vi "Show Panel.vi"(8 "error in (no error)":errorcluster, 11 "View In":refnum<class "View.lvclass">) -> (0 "error out":errorcluster, 3 "View Out":refnum<class "View.lvclass">)   [LabVIEW 2020, in "View.lvclass"]
doc: "Show the front panel of the View."
uses:
  View.lvclass
  C:/Users/anton/Documents/GitHub/Triarc-Framework/source/Framework/Process/Process.lvclass
  Process/Process.lvclass/Process.ctl
  View.lvclass/View.ctl
  Process/Public/Get Lifecycle State.vi
  Process/Protected/Messaging/Request Message.vi
  <vilib>/Utility/error.llb/Clear Errors.vi
  Process/Private/SubVIs/Enqueue Request Message.vi
  <vilib>/Utility/error.llb/Error Cluster From Error Code.vi
  Process/Private/SubVIs/Wait for Response Message.vi
  Process/Process.lvclass
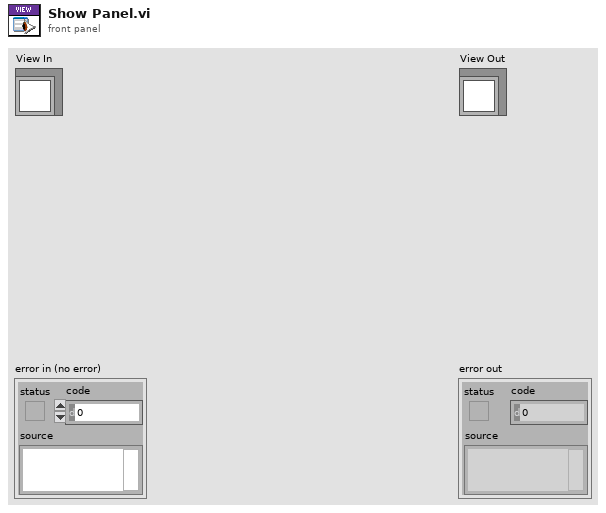
[diagram p1: front panel]
types:
  T1 = typedef "Process.lvclass/Access Mode.ctl" = enum16{"Read", "Request"}
  T2 = enum32{"Invalid", "Standard", "Closed", "Hidden", "Minimized", "Maximized"}
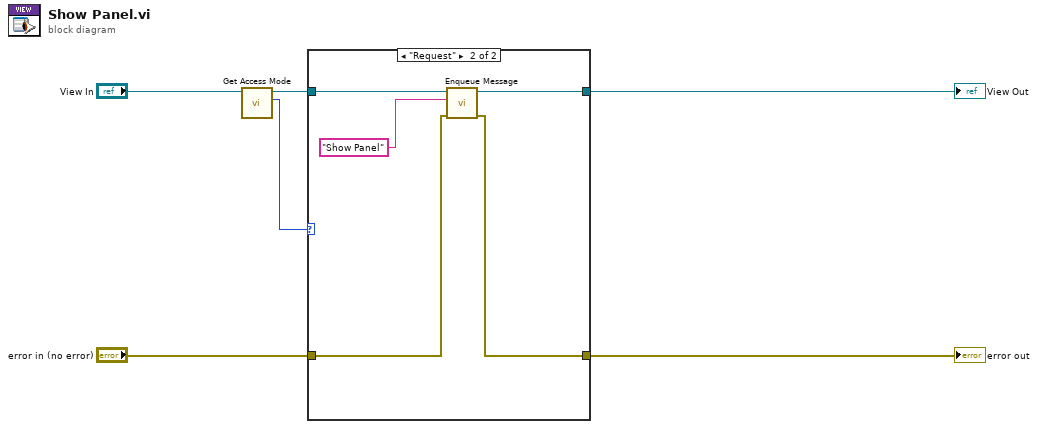
[diagram p0: block diagram]
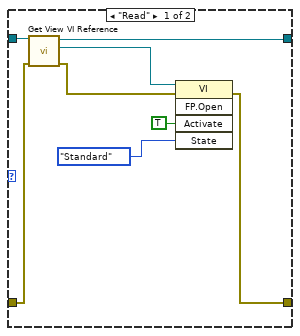
[diagram p2: hidden frame]
diagram:
  n1 = call "Get Access Mode.vi"("Process In"="View In") -> ("Access Mode"=w1:T1, "Process Out"=w2:refnum<class "View.lvclass">)  [unwired: 8 in, 1 out]
  n2 = case shown="\"Request\"" w1 {
    tunnel: [w9 w19] -> w5
    tunnel: [w7 w18] -> w4
    tunnel: "error in (no error)" -> [w8 w17]
    tunnel: w2 -> [w10 w15]
    frame "Read" {
      n3 = call "Get View VI Reference.vi"("error in (no error)"=w8, "UI View In"=w10) -> ("error out"=w11:errorcluster, "View VI Reference"=w14:refnum<vi>, "UI View Out"=w9:refnum<class "View.lvclass">)  [unwired: 7 in]
      n4 = invoke class="VI" method="FP.Open"(reference=w14, error in=w11, "Activate"=TRUE ("Activate?"), "State"=T2."Standard") -> (error out=w7:errorcluster)  [unwired: 1 in, 4 out]
    }
    frame "Request" {
      n5 = call "Enqueue Message.vi"("error in (no error)"=w17, "Message"="Show Panel", "Process In"=w15) -> ("error out"=w18:errorcluster, "Process Out"=w19:refnum<class "View.lvclass">)  [unwired: 7 in]
    }
  }
  "error out" <- w4
  "View Out" <- w5
